vi "BlinkLedExample.vi"   [LabVIEW 2017]
uses:
  <vilib>/Rock Robotics/Network Tables/NT Write Boolean.vi
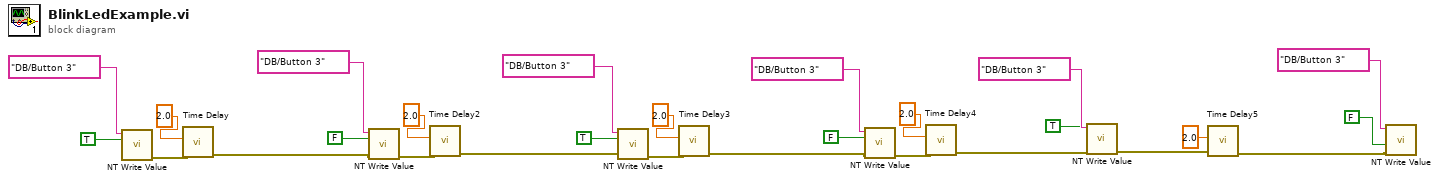
[diagram p0: block diagram]
diagram:
  n1 = call-poly <vilib>:"NT Write Value.vi"("Boolean"=TRUE, "Name"="DB/Button 3") -> ("error out"=w25:errorcluster)  [unwired: 9 in]
  n2 = call "Time Delay"("error in (no error)"=w25, "Delay Time (s)"=2.0) -> ("error out"=w19:errorcluster)  [unwired: 9 in]
  n3 = call-poly <vilib>:"NT Write Value.vi"("error in"=w19, "Boolean"=FALSE, "Name"="DB/Button 3") -> ("error out"=w21:errorcluster)  [unwired: 8 in]
  n4 = call "Time Delay2"("error in (no error)"=w21, "Delay Time (s)"=2.0) -> ("error out"=w9:errorcluster)  [unwired: 9 in]
  n5 = call-poly <vilib>:"NT Write Value.vi"("error in"=w9, "Boolean"=TRUE, "Name"="DB/Button 3") -> ("error out"=w16:errorcluster)  [unwired: 8 in]
  n6 = call "Time Delay3"("error in (no error)"=w16, "Delay Time (s)"=2.0) -> ("error out"=w10:errorcluster)  [unwired: 9 in]
  n7 = call-poly <vilib>:"NT Write Value.vi"("error in"=w10, "Boolean"=FALSE, "Name"="DB/Button 3") -> ("error out"=w12:errorcluster)  [unwired: 8 in]
  n8 = call "Time Delay4"("error in (no error)"=w12, "Delay Time (s)"=2.0) -> ("error out"=w6:errorcluster)  [unwired: 9 in]
  n9 = call-poly <vilib>:"NT Write Value.vi"("error in"=w6, "Boolean"=TRUE, "Name"="DB/Button 3") -> ("error out"=w5:errorcluster)  [unwired: 8 in]
  n10 = call "Time Delay5"("error in (no error)"=w5, "Delay Time (s)"=2.0) -> ("error out"=w1:errorcluster)  [unwired: 9 in]
  n11 = call-poly <vilib>:"NT Write Value.vi"("error in"=w1, "Boolean"=FALSE, "Name"="DB/Button 3") -> ()  [unwired: 8 in, 1 out]
